vi "Module Init.vi"(8 "error in (no error)":errorcluster, 11 "Telemetry Server in":refnum<class "Telemetry Server.lvclass">) -> (0 "error out":errorcluster, 3 "Telemetry Server out":refnum<class "Telemetry Server.lvclass">)   [LabVIEW 2020, in "VolatusTelemetry.lvlib" / "Telemetry Server.lvclass"]
uses:
  Telemetry Server.lvclass
  Publish Group Data.ctl
  lv-protoc/LV-Proto/Message/Message.lvclass
  Telemetry Server.lvclass/Telemetry Server.ctl
  VolatusTelemetry.lvlib
  VolatusConfig/Group Type.ctl
  VolatusConfig/VolatusConfig.lvlib
  IPv4 Endpoint.ctl
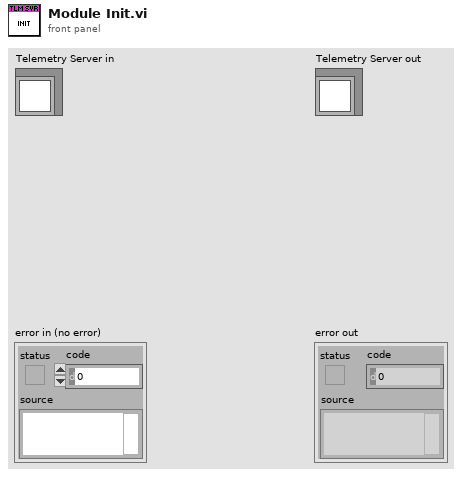
[diagram p1: front panel]
types:
  T1 = typedef "VolatusTelemetry.lvlib/Telemetry Server.lvclass/IPv4 Endpoint.ctl" = cluster{"Address":u32, "Port":u16}
  T2 = typedef "VolatusTelemetry.lvlib/Publish Group Data.ctl" = cluster{"Data Msg":refnum<class "Message.lvclass">, "Group Name":string, "Group Type":T3}
  T3 = typedef "VolatusConfig.lvlib/Group Type.ctl" = enum16{"Double", "Bool", "String"}
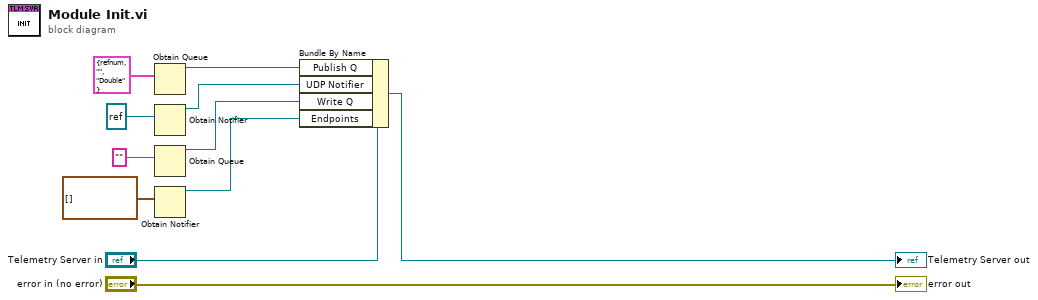
[diagram p0: block diagram]
diagram:
  n1 = Obtain Queue(element data type=T2 {"Data Msg"=refnum, "Group Name"="", "Group Type"=enum."Double"} ("Publish Group Data")) -> (queue out=w7:refnum<queue>)  [unwired: 4 in, 2 out]
  n2 = Obtain Notifier(notification data type=refnum<k16> refnum ("UDP")) -> (notifier out=w5:refnum<notifier>)  [unwired: 3 in, 2 out]
  n3 = Obtain Queue(element data type="") -> (queue out=w4:refnum<queue>)  [unwired: 4 in, 2 out]
  n4 = Obtain Notifier(notification data type=T1[] []) -> (notifier out=w1:refnum<notifier>)  [unwired: 3 in, 2 out]
  n5 = Bundle By Name(cluster="Telemetry Server in", "Publish Q"=w7, "UDP Notifier"=w5, "Write Q"=w4, "Endpoints"=w1) -> (→"Telemetry Server out":refnum<class "Telemetry Server.lvclass">)
  "error out" <- "error in (no error)"
